vi "Main Server.vi"(11 "tCRD in":refnum<class "Open Path CRD.lvclass">) -> (0 "error out":errorcluster)   [LabVIEW 2015]
uses:
  CRD/Open Path CRD.lvclass
  Reusable/Instrument/state.ctl
  Reusable/Session Log/System Log.lvclass
  Reusable/Session APIs/File Access/Config Data/Config Session.ctl
  Reusable/Session APIs/File Access/Config Data/Config Data.lvclass
  Reusable/Session APIs/File Access/Config Data/Config Data.lvclass/Config Data.ctl
  CRD/Data/Open Path Data.lvclass
  CRD/Data/Open Path Data.lvclass/Open Path Data.ctl
  Devices/Alicat/Session Based/Data/Alicat Data.lvclass
  Devices/CR5/Data/CR5 Data.lvclass
  Reusable/CRDS/Data/Cell/CRDS Cell Data.lvclass
  Reusable/CRDS/Data/Cell/CRDS Cell Data.lvclass/CRDS Cell Data.ctl
  Devices/CR5/Data/CR5 Data.lvclass/CR5 Data.ctl
  Reusable/Session Log/System Log.lvclass/System Log.ctl
  Reusable/Instrument/Instrument.lvclass/Instrument.ctl
  Devices/CR5/Data/Accessors/Read Balance.vi
  Devices/CR5/Data/Accessors/Read flag.vi
  Devices/CR5/Data/Accessors/Read mirror flag.vi
  Devices/CR5/Data/Accessors/Read PWM.vi
  Devices/CR5/Data/Accessors/Read Tamb.vi
  Devices/CR5/Data/Accessors/Read Tboard.vi
  Devices/CR5/Data/Accessors/Read Tmirror.vi
  Reusable/CRDS/Data/Cell/Read extParam.vi
  CRD/Data/Read Alicat Data.vi
  CRD/Data/Accessors/Read CR5.vi
  CRD/Data/Accessors/Read Heated Line Temp.vi
  CRD/Data/Accessors/Read Thermistor Data.vi
  CRD/Data/Accessors/Read u.vi
  CRD/Data/Accessors/Read VaisalaDuct.vi
  CRD/Data/Accessors/Read VaisalaOutside.vi
  CRD/Data/Accessors/Read Pressure.vi
  Reusable/Session APIs/File Access/Config Data/Accessors/Write Cfg Path.vi
  Reusable/Session APIs/File Access/Config Data/Accessors/Read Ref.vi
  Reusable/Session Log/Accessors/Write Main Path.vi
  Reusable/Instrument/Write Log Session.vi
  <vilib>/Utility/tcp.llb/UDP Multicast Write-Only Open.vi
  <vilib>/Utility/config.llb/Read Key (Boolean).vi
  <vilib>/Utility/config.llb/Read Key (I32).vi
  <vilib>/Utility/config.llb/Read Key (String).vi
  <vilib>/Utility/config.llb/Read Key (Path).vi
  Reusable/Data/Read measTime.vi
  Reusable/CRDS/Data/Main/Read CellData.vi
  Reusable/CRDS/Data/Main/Read filter.vi
  Reusable/Instrument/Instrument.lvclass
  <userlib>/_Session Fwk/Session - Root.lvclass
  Reusable/File IO/File Utilities.lvlib
  <vilib>/nisyscfg/nisyscfg.lvlib
  <vilib>/Utility/config.llb/NI_LVConfig.lvlib
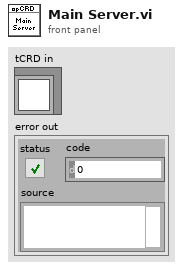
[diagram p1: front panel]
types:
  T1 = typedef "Config Data.lvclass/Config Session.ctl" = refnum<data-value>
  T2 = typedef "Instrument.lvclass/state.ctl" = enum8{"Configure", "Acquire", "Wait", "Quit", "Handle Error", "NOOP"}
  T3 = typedef "Session - Root.lvclass/Session Handle.ctl" = refnum<data-value>
  T4 = typedef "NI_LVConfig.lvlib/Config Data RefNum.ctl" = refnum<k1>
  T5 = typedef "extparam.ctl" = cluster{"Tau":sgl, "Tau0cor":sgl, "ext":sgl, "extCorr":sgl, "stdevTau":sgl, "eTau":sgl, "taucorr":sgl, "Tau0":sgl, "max":sgl}
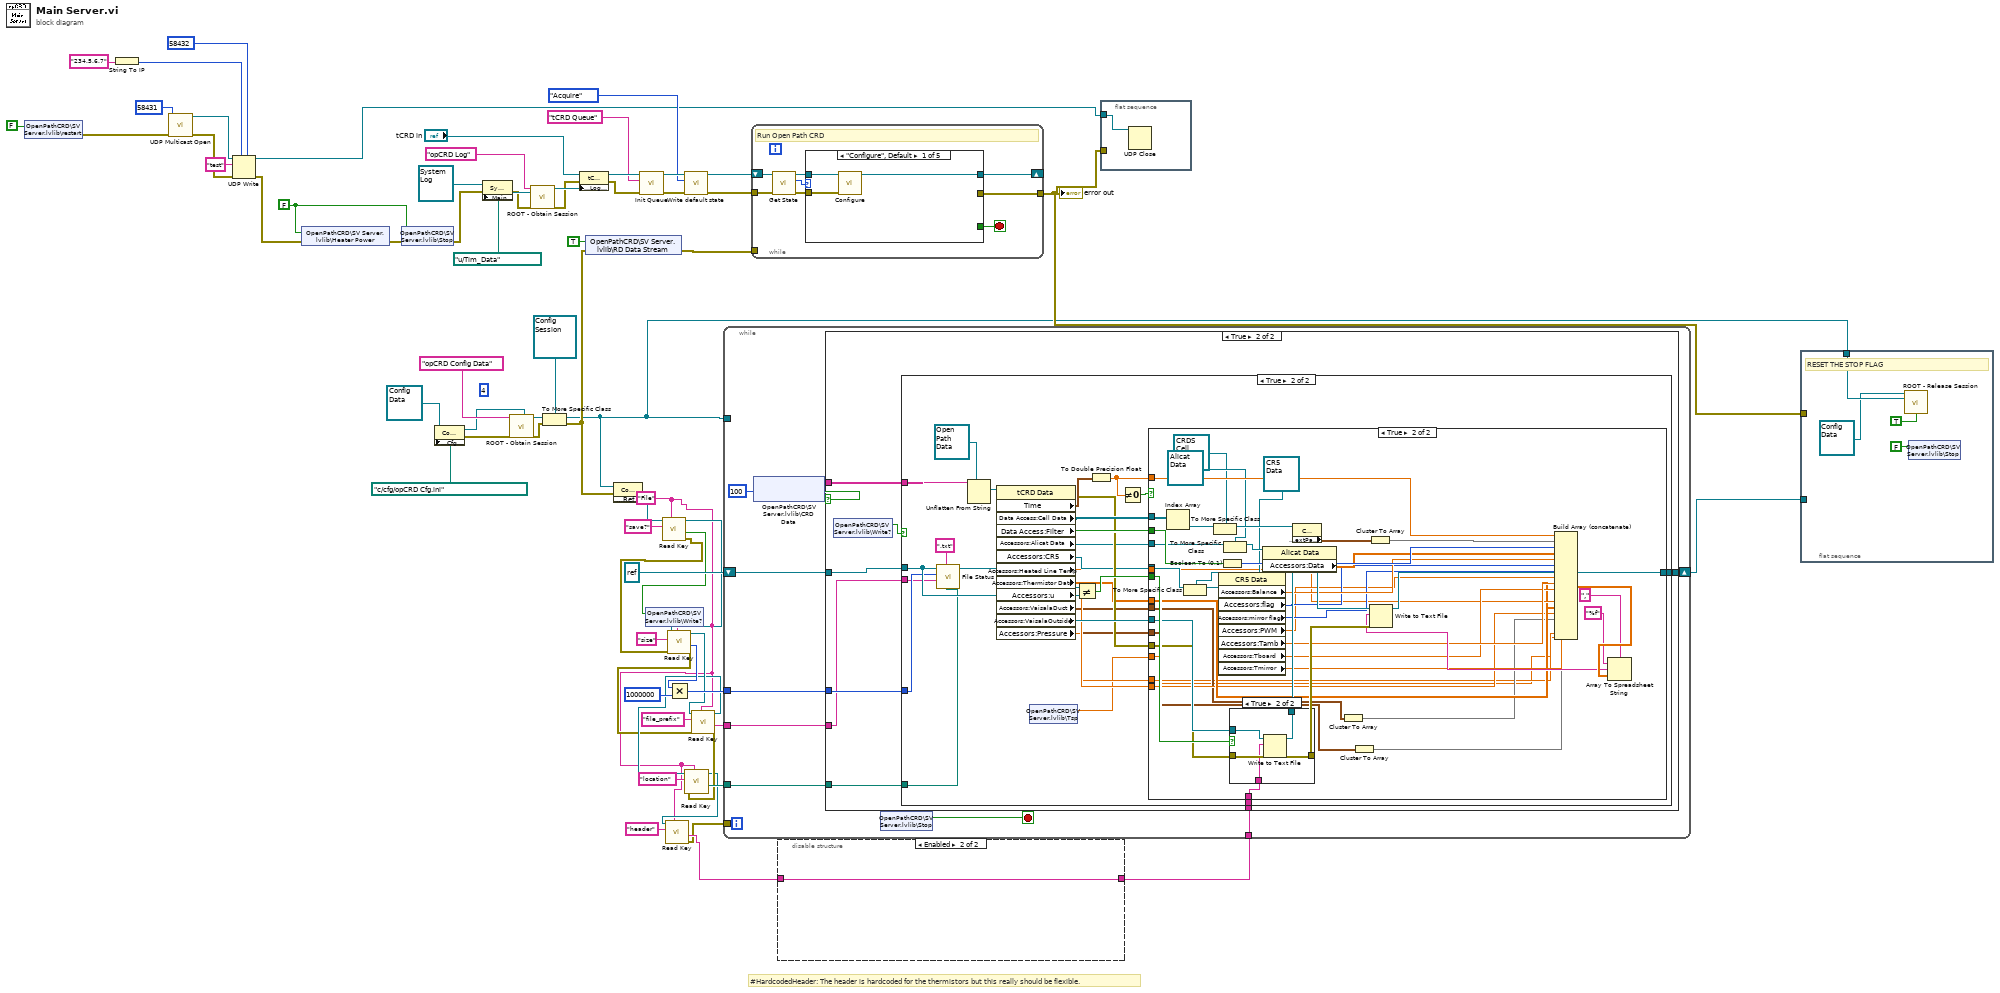
[diagram p0: block diagram]
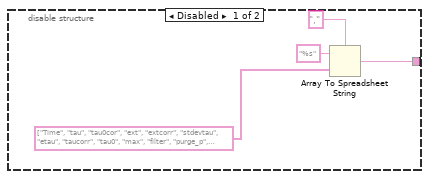
[diagram p2: hidden frame]
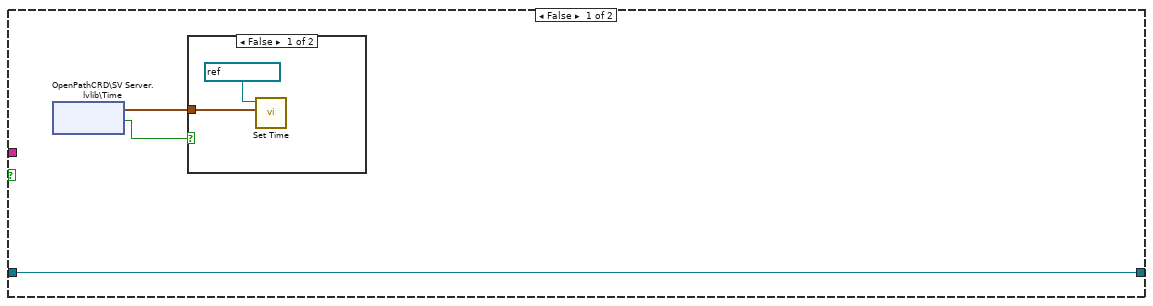
[diagram p3: hidden frame]
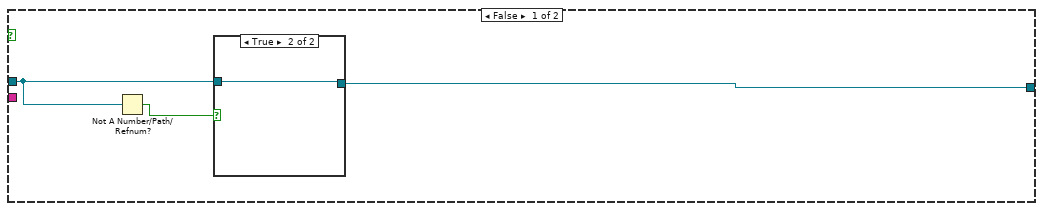
[diagram p5: hidden frame]
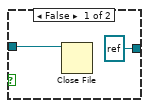
[diagram p6: hidden frame]
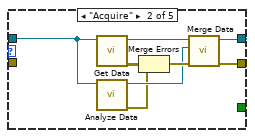
[diagram p9: hidden frame]
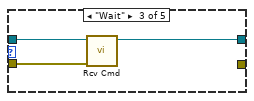
[diagram p10: hidden frame]
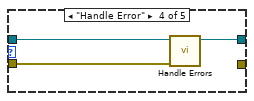
[diagram p11: hidden frame]
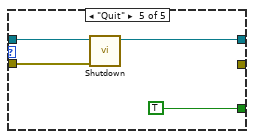
[diagram p12: hidden frame]
diagram:
  w5 = "File" ("section")
  (unwired) 4
  w45 = FALSE ("Stop")
  # "#HardcodedHeader: The header is hardcoded for the thermistors but this really should be flexible."
  n1 = shared-variable "OpenPathCRD\\SV Server.lvlib\\restart"(FALSE ("restart")) -> (error out=w33:errorcluster)  [unwired: 1 in]
  n2 = String To IP(1:"234.5.6.7" ("name")) -> (0:w40:u32)
  n3 = call-poly <vilib>:"UDP Multicast Open.vi"("error in (no error)"=w33, "port"=u16 58431) -> ("error out"=w41:errorcluster, "connection ID"=w42:refnum<k16>)  [unwired: 8 in]
  n4 = UDP Write(address=w40, port or service name=u16 58432, connection ID=w42, data in="test", 8:w41) -> (error out=w38:errorcluster, 3:w37:refnum<k16>)  [unwired: 1 in]
  n5 = shared-variable "OpenPathCRD\\SV Server.lvlib\\Heater Power"(w45, error in=w38) -> (error out=w46:errorcluster)
  n6 = shared-variable "OpenPathCRD\\SV Server.lvlib\\Stop"(w45, error in=w46) -> (error out=w49:errorcluster)
  n7 = property class="Config Data"(reference=refnum<class "Config Data.lvclass"> refnum ("Config Data"), "Accessors:Cfg Path"=path "c:/cfg/opCRD Cfg.ini" ("Path")) -> (reference out=w27:refnum<class "Config Data.lvclass">, error out=w28:errorcluster)  [unwired: 1 in]
  n8 = property class="Sys Log"(reference=refnum<class "System Log.lvclass"> refnum ("Sys Log"), error in=w49, "Accessors:Main Path"=path "u:/Tim_Data" ("RD Data Path")) -> (reference out=w59:refnum<class "System Log.lvclass">, error out=w58:errorcluster)
  n9 = call <userlib>:"ROOT - Obtain Session.vi"("Session Name ()"="opCRD Config Data", "OBJ - Session"=w27, "error in (no error)"=w28) -> ("Session Handle"=w26:T3, "error out"=w25:errorcluster)  [unwired: 10 in, 1 out]
  n10 = call <userlib>:"ROOT - Obtain Session.vi"("Session Name ()"="opCRD Log", "OBJ - Session"=w59, "error in (no error)"=w58) -> ("Session Handle"=w56:T3, "error out"=w55:errorcluster)  [unwired: 10 in, 1 out]
  n11 = To More Specific Class(target class=T1 refnum ("Session Handle"), reference=w26, error in=w25) -> (specific class reference=w2:T1, error out=w24:errorcluster)
  n12 = property class="tCRD"(reference="tCRD in", error in=w55, "Accessors:Log Session"=w56) -> (reference out=w68:refnum<class "Open Path CRD.lvclass">, error out=w53:errorcluster)
  n13 = shared-variable "OpenPathCRD\\SV Server.lvlib\\RD Data Stream"(TRUE ("RD Data Stream"), error in=w24) -> (error out=w51:errorcluster)
  n14 = property class="Config Data"(reference=w2, error in=w24) -> ("Accessors:Ref"=w23:T4)  [unwired: 2 out]
  n15 = call "Init Queue.vi"("error in"=w53, "queue_name"="tCRD Queue", "Instrument in"=w68) -> ("error out"=w66:errorcluster, "Instrument out"=w65:refnum<class "Open Path CRD.lvclass">)  [unwired: 7 in]
  n16 = call-poly <vilib>:"Read Key.vi"("section"=w5, "key"="save?", "refnum"=w23) -> ("error out"=w15:errorcluster, "value"=w21:bool, "refnum out"=w20:T4)  [unwired: 5 in, 1 out]
  n17 = shared-variable "OpenPathCRD\\SV Server.lvlib\\Write?"(w21) -> ()  [unwired: 1 in, 1 out]
  n18 = call-poly <vilib>:"Read Key.vi"("section"=w5, "error in (no error)"=w15, "key"="size", "refnum"=w20) -> ("error out"=w8:errorcluster, "value"=w18:i32, "refnum out"=w14:T4)  [unwired: 4 in, 1 out]
  n19 = Multiply(x=w18, y=1000000) -> (x*y=w16:i32)
  n20 = call "Write default state.vi"("error in (no error)"=w66, "instr state"=state."Acquire", "Instrument in"=w65) -> ("error out"=w47:errorcluster, "Instrument out"=w64:refnum<class "Open Path CRD.lvclass">)  [unwired: 7 in]
  n21 = call-poly <vilib>:"Read Key.vi"("section"=w5, "error in (no error)"=w8, "key"="file_prefix", "refnum"=w14) -> ("error out"=w7:errorcluster, "value"=w12:string, "refnum out"=w11:T4)  [unwired: 4 in, 1 out]
  n22 = call-poly <vilib>:"Read Key.vi"("section"=w5, "error in (no error)"=w7, "key"="location", "refnum"=w11) -> ("value"=w9:path, "refnum out"=w6:T4)  [unwired: 4 in, 2 out]
  n23 = call-poly <vilib>:"Read Key.vi"("section"=w5, "key"="header", "refnum"=w6) -> ("error out"=w1:errorcluster, "value"=w3:string)  [unwired: 5 in, 2 out]
  n24 = while "Acquisition" {
    tunnel: w47 -> [w76]
    shift-right: [w73] -> _
    shift-left: w64 -> [w75]
    tunnel: [w72] -> w36
    tunnel: w51 -> [_]
    stop <- w74 stop-if-true
    # "Run Open Path CRD"
    n25 = call "Get State.vi"("error in"=w76, "Instrument in"=w75) -> ("error out"=w69:errorcluster, "default state"=w71:T2, "Instrument out"=w70:refnum<class "Open Path CRD.lvclass">)  [unwired: 7 in]
    n26 = case shown="\"Configure\", Default" w71 {
      tunnel: w70 -> [w79 w86 w89 w93 w96]
      tunnel: w69 -> [w78 _ w88 w92 w95]
      tunnel: [_ _ _ _ TRUE] -> w74
      tunnel: [w77 w87 w90 w91 w94] -> w73
      tunnel: [_ w85 _ _ _] -> w72
      frame "Configure", Default {
        n27 = call-dynamic "Configure.vi"("error in"=w78, "tCRD in"=w79) -> ("tCRD out"=w77:refnum<class "Open Path CRD.lvclass">)  [unwired: 8 in, 1 out]
      }
      frame "Acquire" {
        n28 = call-dynamic "Get Data.vi"("tCRD in"=w86) -> ("error out"=w81:errorcluster, "tCRD out"=w84:refnum<class "Open Path CRD.lvclass">)  [unwired: 9 in]
        n29 = call-dynamic "Analyze Data.vi"("tCRD in"=w86) -> ("error out"=w80:errorcluster, "tCRD out"=w82:refnum<class "Open Path CRD.lvclass">)  [unwired: 9 in]
        n30 = Merge Errors(w81, w80) -> (w83:errorcluster)
        n31 = call-dynamic "Merge Data.vi"("error in"=w83, "Analyzed"=w82, "Acquired"=w84) -> ("error out"=w85:errorcluster, "tCRD out"=w87:refnum<class "Open Path CRD.lvclass">)  [unwired: 7 in]
      }
      frame "Wait" {
        n32 = call-dynamic "Rcv Cmd.vi"("error in"=w88, "tCRD in"=w89) -> ("tCRD out"=w90:refnum<class "Open Path CRD.lvclass">)  [unwired: 8 in, 1 out]
      }
      frame "Handle Error" {
        n33 = call-dynamic "Handle Errors.vi"("error in"=w92, "tCRD in"=w93) -> ("tCRD out"=w91:refnum<class "Open Path CRD.lvclass">)  [unwired: 7 in, 2 out]
      }
      frame "Quit" {
        n34 = call-dynamic "Shutdown.vi"("error in"=w95, "tCRD in"=w96) -> ("tCRD out"=w94:refnum<class "Open Path CRD.lvclass">)  [unwired: 8 in, 1 out]
      }
    }
  }
  "error out" <- w36
  n35 = disable-structure shown="Enabled" {
    disable-tunnel: [w98 w102] -> w50
    disable-tunnel: w3 -> [_ w102]
    frame Disabled {
      n36 = Array To Spreadsheet String(delimiter (Tab)=",", array=string[] ["Time", "tau", "tau0cor", "ext", "extcorr", "stdevtau", "etau", "taucorr", "tau0", "max", "filter", "purge_p", "purge_T", "purge_Q", "purge_Q0", "purge_Qsp", "cr5_balance", "cr5_flag", "cr5_mirror_flag", "cr5_pwm", "cr5_Tamb", "cr5_Tboard", "cr5_Tmirror", "Theatedline", "Thermistor_1", "Thermistor_2", "u", "vaisala_RH_duct", "vaisala_T_duct", "vaisala_RH_ambient", "vaisala_T_ambient", "Pressure", "T_heated_SP"], 3:"%s" ("format string")) -> (spreadsheet string=w98:string)
    }
    frame Enabled {
    }
  }
  n37 = while {
    shift-right: [w107] -> w48
    shift-left: refnum<file> refnum ("fileRefIn") -> [w108]
    tunnel: w50 -> [w106]
    tunnel: w2 -> [_]
    tunnel: w16 -> [w105]
    tunnel: w12 -> [w104]
    tunnel: w9 -> [w103]
    tunnel: w1 -> [_]
    stop <- w112 stop-if-true
    n38 = shared-variable "OpenPathCRD\\SV Server.lvlib\\CRD Data"(100 ("ms timeout (0)")) -> (w109:string, w110:bool)  [unwired: 1 in, 1 out]
    n39 = case shown="True" w110 {
      tunnel: w109 -> [_ w125]
      tunnel: w108 -> [w115 w124]
      tunnel: [w115 w123] -> w107
      tunnel: w106 -> [_ w121]
      tunnel: w105 -> [_ w120]
      tunnel: w104 -> [_ w119]
      tunnel: w103 -> [_ w118]
      frame False {
        n40 = shared-variable "OpenPathCRD\\SV Server.lvlib\\Time"() -> (w114:timestamp, w113:bool)  [unwired: 2 in, 1 out]
        n41 = case shown="False" w113 {
          tunnel: w114 -> [w117 _]
          frame False {
            n42 = call <vilib>:"Set Time.vi"("Time"=w117, "Session in (localhost)"=refnum<k21> "localhost") -> ()  [unwired: 6 in, 4 out]
          }
          frame True {
          }
        }
      }
      frame True {
        n43 = shared-variable "OpenPathCRD\\SV Server.lvlib\\Write?"() -> (w122:bool)  [unwired: 1 in, 1 out]
        n44 = case shown="True" w122 {
          tunnel: w125 -> [_ w158]
          tunnel: w124 -> [w127 w151]
          tunnel: [w126 w146] -> w123
          tunnel: w121 -> [_ w144]
          tunnel: w120 -> [_ w134]
          tunnel: w119 -> [_ w133]
          tunnel: w118 -> [_ w132]
          frame False {
            n45 = Not A Number/Path/Refnum?(number/path/refnum=w127) -> (NaN/Path/Refnum?=w128:bool)
            n46 = case shown="True" w128 {
              tunnel: w127 -> [w130 w131]
              tunnel: [refnum<file> refnum ("refnum out") w131] -> w126
              frame False {
                n47 = Close File(refnum=w130) -> ()  [unwired: 1 in, 2 out]
              }
              frame True {
              }
            }
          }
          frame True {
            n48 = call "File Status.vi"("Data Path"=w132, "ext"=".txt", "prefix"=w133, "fSize"=w134, "fileRefIn"=w151) -> ("fileRefOut"=w147:refnum<file>)  [unwired: 5 in, 1 out]
            n49 = Unflatten From String(type=refnum<class "Open Path Data.lvclass"> refnum ("tCRD Data"), binary string=w158) -> (value=w156:refnum<class "Open Path Data.lvclass">)  [unwired: 3 in, 2 out]
            n50 = property class="tCRD Data"(reference=w156) -> (error out=w145:errorcluster, "Time"=w154:timestamp, "Data Access:Cell Data"=w155:refnum<class "CRDS Cell Data.lvclass">[], "Data Access:Filter"=w153:bool, "Accessors:Alicat Data"=w143:refnum<class "Alicat Data.lvclass">, "Accessors:CR5"=w142:refnum<class "CR5 Data.lvclass">, "Accessors:Heated Line Temp"=w141:dbl, "Accessors:Thermistor Data"=w140:dbl[], "Accessors:u"=w139:sgl, "Accessors:VaisalaDuct"=w138:cluster{"RH":sgl, "T":sgl}, "Accessors:VaisalaOutside"=w137:cluster{"RH":sgl, "T":sgl}, "Accessors:Pressure"=w136:dbl)  [unwired: 1 in, 1 out]
            n51 = shared-variable "OpenPathCRD\\SV Server.lvlib\\Tsp"() -> (w135:dbl)  [unwired: 1 in, 1 out]
            n52 = Not Equal?(x=w147, y=w151) -> (x != y?=w148:bool)
            n53 = To Double Precision Float(number=w154) -> (double precision float=w150:dbl)
            n54 = Not Equal To 0?(x=w150) -> (x != 0?=w149:bool)
            n55 = case shown="True" w149 {
              tunnel: w155 -> [_ w202]
              tunnel: w150 -> [_ w197]
              tunnel: w153 -> [_ w196]
              tunnel: w148 -> [_ w194]
              tunnel: w147 -> [w159 w193]
              tunnel: [w159 w189] -> w146
              tunnel: w145 -> [_ w192]
              tunnel: w144 -> [_ w184]
              tunnel: w143 -> [_ w183]
              tunnel: w142 -> [_ w179]
              tunnel: w141 -> [_ w169]
              tunnel: w140 -> [_ w168]
              tunnel: w139 -> [_ w167]
              tunnel: w138 -> [_ w166]
              tunnel: w137 -> [_ w164]
              tunnel: w136 -> [_ w161]
              tunnel: w135 -> [_ w160]
              frame False {
              }
              frame True {
                n56 = Index Array(array=w202) -> (element=w201:refnum<class "CRDS Cell Data.lvclass">)  [unwired: 1 in]
                n57 = To More Specific Class(target class=refnum<class "CR5 Data.lvclass"> refnum ("CR5 Data"), reference=w179) -> (specific class reference=w177:refnum<class "CR5 Data.lvclass">)  [unwired: 1 in, 1 out]
                n58 = To More Specific Class(target class=refnum<class "CRDS Cell Data.lvclass"> refnum ("CRDS Cell"), reference=w201) -> (specific class reference=w200:refnum<class "CRDS Cell Data.lvclass">)  [unwired: 1 in, 1 out]
                n59 = property class="CR5 Data"(reference=w177) -> ("Accessors:Balance"=w176:dbl, "Accessors:flag"=w175:i32, "Accessors:mirror flag"=w174:i32, "Accessors:PWM"=w173:dbl, "Accessors:Tamb"=w172:dbl, "Accessors:Tboard"=w171:dbl, "Accessors:Tmirror"=w170:dbl)  [unwired: 1 in, 2 out]
                n60 = Boolean To (0,1)(Boolean=w196) -> (0, 1=w195:i16)
                n61 = To More Specific Class(target class=refnum<class "Alicat Data.lvclass"> refnum ("Alicat Data"), reference=w183) -> (specific class reference=w181:refnum<class "Alicat Data.lvclass">)  [unwired: 1 in, 1 out]
                n62 = case shown="True" w194 {
                  tunnel: w193 -> [w204 w209]
                  tunnel: [w204 w208] -> w190
                  tunnel: w192 -> [w203 w207]
                  tunnel: [w203 w206] -> w191
                  tunnel: w184 -> [_ w205]
                  frame False {
                  }
                  frame True {
                    n63 = Write to Text File(file (use dialog)=w209, text=w205, error in=w207) -> (refnum out=w208:refnum<file>, error out=w206:errorcluster)  [unwired: 1 in, 1 out]
                  }
                }
                n64 = property class="Alicat Data"(reference=w181) -> ("Accessors:Data"=w180:sgl[])  [unwired: 1 in, 2 out]
                n65 = property class="CRDS Cell"(reference=w200) -> ("Data Access:extParam"=w199:T5)  [unwired: 1 in, 2 out]
                n66 = Cluster To Array(cluster=w166) -> (array=w165:sgl[])
                n67 = Cluster To Array(cluster=w164) -> (array=w163:sgl[])
                n68 = Cluster To Array(cluster=w199) -> (array=w198:sgl[])
                n69 = Build Array (concatenate)(w197, w198, w195, w180, w176, w175, w174, w173, w172, w171, w170, w169, w168, w167, w165, w163, w161, w160) -> (w188:dbl[])
                n70 = Array To Spreadsheet String(delimiter (Tab)=",", array=w188, 3:"%f" ("format string")) -> (spreadsheet string=w185:string)
                n71 = Write to Text File(file (use dialog)=w190, text=w185, error in=w191) -> (refnum out=w189:refnum<file>)  [unwired: 1 in, 2 out]
              }
            }
          }
        }
      }
    }
    n72 = shared-variable "OpenPathCRD\\SV Server.lvlib\\Stop"() -> (w112:bool)  [unwired: 1 in, 1 out]
  }
  n73 = flat-sequence {
    tunnel: w37 -> [w210]
    tunnel: w36 -> [_]
    frame #0 {
      n74 = UDP Close(connection ID=w210) -> ()  [unwired: 1 in, 2 out]
    }
  }
  n75 = flat-sequence {
    tunnel: w48 -> [_]
    tunnel: w36 -> [_]
    tunnel: w2 -> [w213]
    frame #0 {
      # "RESET THE STOP FLAG"
      n76 = call <userlib>:"ROOT - Release Session.vi"("OBJ - Session in"=refnum<class "Config Data.lvclass"> refnum ("Config Data"), "Session Handle in"=w213, "force destroy? (F)"=TRUE) -> ()  [unwired: 11 in, 2 out]
      n77 = shared-variable "OpenPathCRD\\SV Server.lvlib\\Stop"(FALSE ("Stop")) -> ()  [unwired: 1 in, 1 out]
    }
  }
